vi "About.vi"(0 "MLA":refnum<class "MLA.lvclass">, 5 "error in (no error)":errorcluster) -> (14 "MLA":refnum<class "MLA.lvclass">, 15 "Cancelled?":bool, 19 "error out":errorcluster)   [LabVIEW 2017, in "MLA.lvclass"]
doc: "Use this template to create a dialog box with event handling."
uses:
  MLA.lvclass
  <vilib>/Platform/browser.llb/Open URL in Default Browser (string).vi
panel:
  out "Version":string caption="Test SW Revision:"
  out "AppName":string caption="App Name"
  in  "S5Link":bool
  out "Revision History":string
  in  "OK":bool
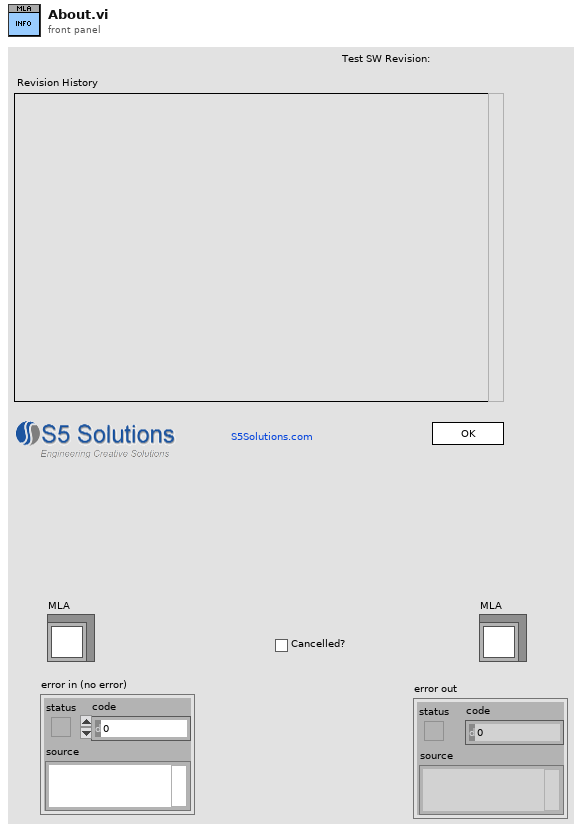
[diagram p1: front panel]
types:
  T1 = typedef "MLA.lvclass/ObjectAttributes.ctl" = cluster{"App Name":string, "App Version":string, "Revision History":string, "Log File Path":path, "Config INI File":path, "Config Path":path, "Log Archive Path":path, "Msg Q's":refnum<queue>[], "VI":refnum<vi>, "ErrLog":refnum<class "ErrorLog.lvclass">}
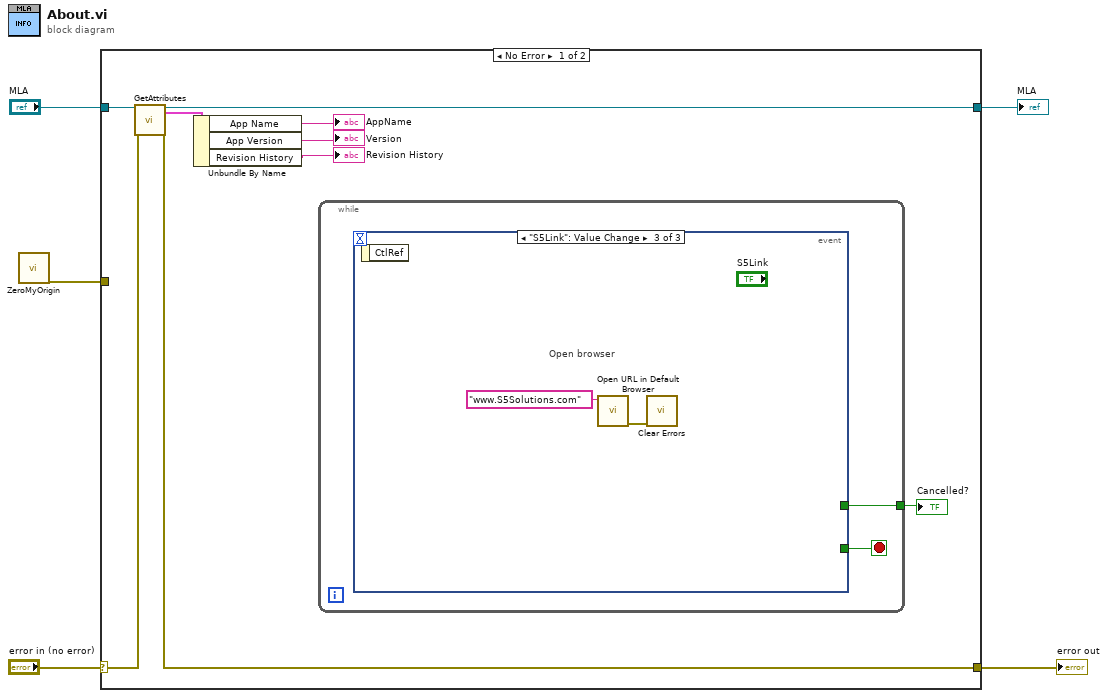
[diagram p0: block diagram]
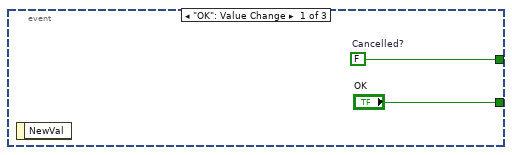
[diagram p2: hidden frame]
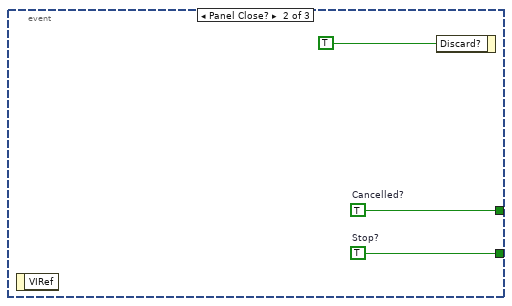
[diagram p3: hidden frame]
diagram:
  n1 = call "ZeroMyOrigin.vi"() -> ("error out"=w1:errorcluster)  [unwired: 19 in]
  n2 = case shown="No Error" "error in (no error)" {
    selector: "error in (no error)" -> [w13 w25]
    tunnel: [w12 w25] -> w4
    tunnel: "MLA" -> [w11 w24]
    tunnel: [w10 w24] -> w2
    tunnel: w1 -> [_ _]
    frame No Error {
      n3 = call "GetAttributes.vi"("MLA"=w11, "error in (no error)"=w13) -> ("MLA"=w10:refnum<class "MLA.lvclass">, "Data"=w9:T1, "error out"=w12:errorcluster)  [unwired: 14 in, 1 out]
      n4 = Unbundle By Name(w9) -> ("App Name"=→"AppName":string, "App Version"=→"Version":string, "Revision History"=→"Revision History":string)
      n5 = while {
        tunnel: [w15] -> w14
        stop <- w16 stop-if-true
        n6 = event shown="[2] \"S5Link\": Value Change" {
          selector: _ -> [_ _ _]
          dyn-events: _ -> [_ _ _]
          timeout: _ -> [_ _ _]
          tunnel: ["OK" w20 _] -> w16
          tunnel: [w18 w19 _] -> w15
          event "OK": Value Change {
            w18 = FALSE  # Cancelled?
            n7 = event-data() -> ()  [unwired: 1 in, 1 out]
          }
          event Panel Close? {
            w19 = TRUE  # Cancelled?
            w20 = TRUE  # Stop?
            n8 = event-data() -> ()  [unwired: 1 in, 1 out]
            n9 = event-data("Discard?"=TRUE) -> ()  [unwired: 1 in, 1 out]
          }
          event "S5Link": Value Change {
            # "Open browser"
            n10 = event-data() -> ()  [unwired: 1 in, 1 out]
            n11 = call-poly <vilib>:"Open URL in Default Browser.vi"("URL"="www.S5Solutions.com") -> ("error out"=w23:errorcluster)  [unwired: 5 in, 1 out]
            n12 = call <vilib>:"Clear Errors.vi"("error in (no error)"=w23) -> ()  [unwired: 5 in, 2 out]
          }
        }
      }
      "Cancelled?" <- w14
    }
    frame Error {
    }
  }
  "error out" <- w4
  "MLA" <- w2
